vi "Time Estimate.vi"(8 "error in (no error)":errorcluster, 10 "Points":dbl, 11 "PC Reader in":refnum<class "PC Reader.lvclass">) -> (0 "error out":errorcluster, 2 "time":dbl[unit], 3 "PC Reader out":refnum<class "PC Reader.lvclass">)   [LabVIEW 2015, in "PC Reader.lvclass"]
uses:
  PC Reader.lvclass
  Reader/Reader.lvclass
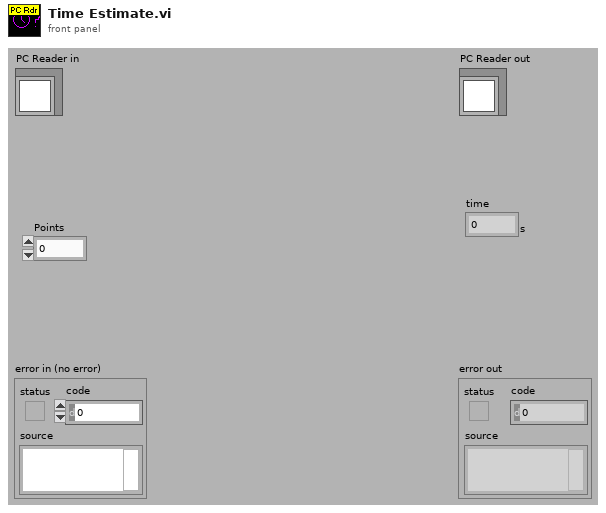
[diagram p1: front panel]
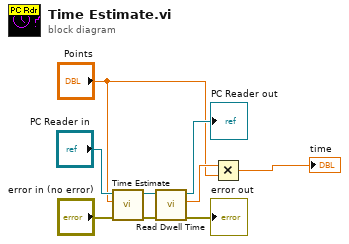
[diagram p0: block diagram]
diagram:
  n1 = call-parent "Time Estimate.vi"("error in (no error)"="error in (no error)", "Points"="Points", "Reader in"="PC Reader in") -> ("error out"=w5:errorcluster, "Reader out"=w6:refnum<class "PC Reader.lvclass">)  [unwired: 6 in, 1 out]
  n2 = call-dynamic "Read Dwell Time.vi"("error in (no error)"=w5, "Reader.lvclass in"=w6) -> ("error out"=→"error out":errorcluster, "Dwell Time"=w3:dbl[unit], "Reader.lvclass out"=→"PC Reader out":refnum<class "PC Reader.lvclass">)  [unwired: 6 in, 1 out]
  n3 = Multiply(x=w3, y="Points") -> (x*y=→"time":dbl[unit])
